vi "T03 - вкл-откл каналов(Base Functions).vi"() -> ()   [LabVIEW 2009]
uses:
  Z210/Z210 CTL Lib.llb/Z210 CTL ADC Inputs Status.ctl
  Z210/Z210 CTL Lib.llb/Z210 CTL ADC Channel Type.ctl
  Z210/Z210 CTL Lib.llb/Z210 CTL DAC Inputs Status.ctl
  Z210/Z210 CTL Lib.llb/Z210 CTL ADC or DAC Function.ctl
  Instance           3 46Saved   T03 - вкл-откл каналов(Base Functions) .vi
  Z210/Z210 Base Functions.llb/Z210 CHANNEL AD Set On/Off.vi
  Z210/Z210 Base Functions.llb/Z210 CHANNEL AD Get On/Off Status.vi
  <vilib>/Utility/error.llb/DialogType.ctl
panel:
  out "Leads Status DAC":T1
  out "Leads Status ADC":T2
  out "leadsAmount DAC":i32
  out "leadsAmount ADC":i32
  out "error out":errorcluster {"code" format="%x"}
  out "workChannel DAC":i32
  out "workChannel ADC":i32
  # "Пример не очень правильной работы с \"канальными\" функциями. Более правильная в T04.\n\na. Выводы АЦП образуют канал работающий в дифференциальном режиме только парами четный-нечетный (нумерацию с 0).\nНапример выводы №0 и №1 могут работать в дифференциальном режиме, а №1 и №2 — нет.\nb. Если опросить состояние выводов АЦП, работающих в дифференциальном режиме, то будет как на Рис 1. Вне зависимости\nбыл ли включен нечетный канал явно, он будет отмечен как выключенный (ср. T03 и T04).\nс. При использовании Base Function легко допустить ошибку (см. п3)."
  # "Рис. 1"
  # "нельзя проверить правильно ли работает этот пример пока нет сбора данных."
  # "Общее число каналов в устройстве"
  # "Количество включенных каналов"
  # "Программа отключает все каналы (подтверждение),\nзатем предлагает включить последовательно несколько\nсначала синфазных, а затем дифференциальных каналов\n\n1. Синфазные каналы включаются корректно в любом количестве\nне превышающем число выводов.\n2. Если количестов синфазных каналов четное — дифф тоже\nвключаются норм.\n3. Внимание! Попытка включить в синфазном режиме 0й и\nв дифференциальном 1й и 2й выводы не приведет к ошибке,\nкак можно было бы ожидать. Вместо этого дифференциальный \nканал образуют 0й и 1й выводы, а состояние 2го зависит\nот того как включать, и что с ним было до того. (ср. T04)"
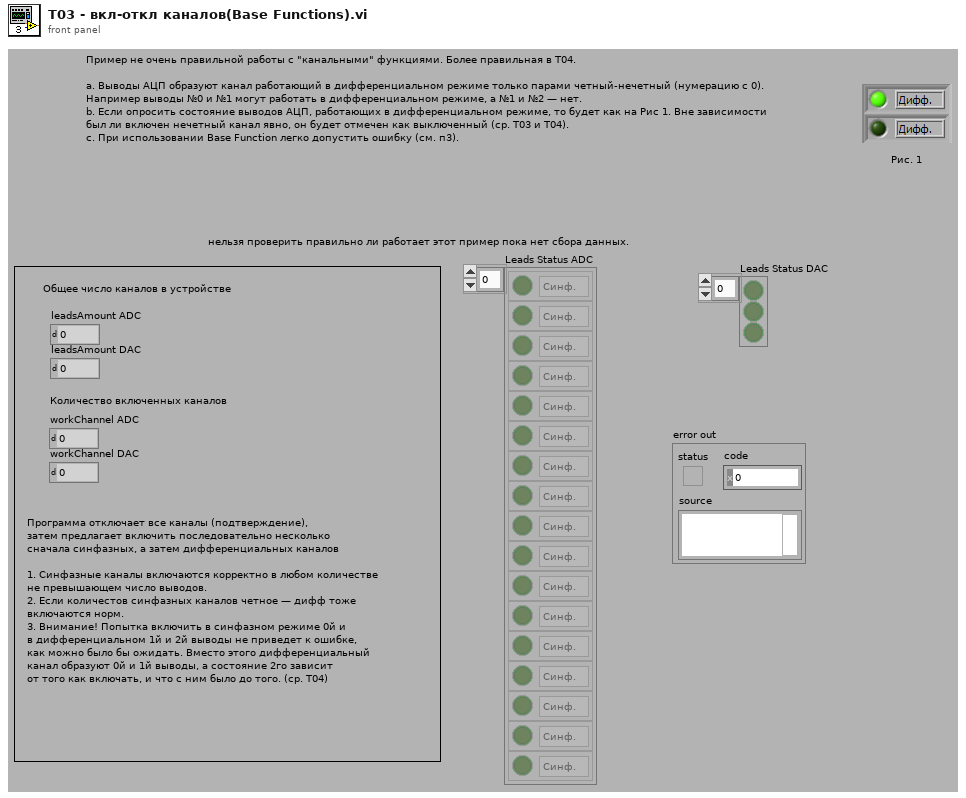
[diagram p1: front panel]
types:
  T1 = typedef "Z210 CTL DAC Inputs Status.ctl" = bool[]
  T2 = typedef "Z210 CTL ADC Inputs Status.ctl" = cluster{"isEnabled?":bool, "ADCchType":T3}[]
  T3 = typedef "Z210 CTL ADC Channel Type.ctl" = enum16{"Синф.", "Дифф."}
  T4 = typedef "Z210 CTL ADC or DAC Function.ctl" = enum16{"АЦП", "ЦАП", "Both"}
  T5 = typedef "Z210 CTL Unit Data .ctl" = cluster{"typeDevice":i32, "numberDSP":i32}
  T6 = typedef "DialogType.ctl" = u16
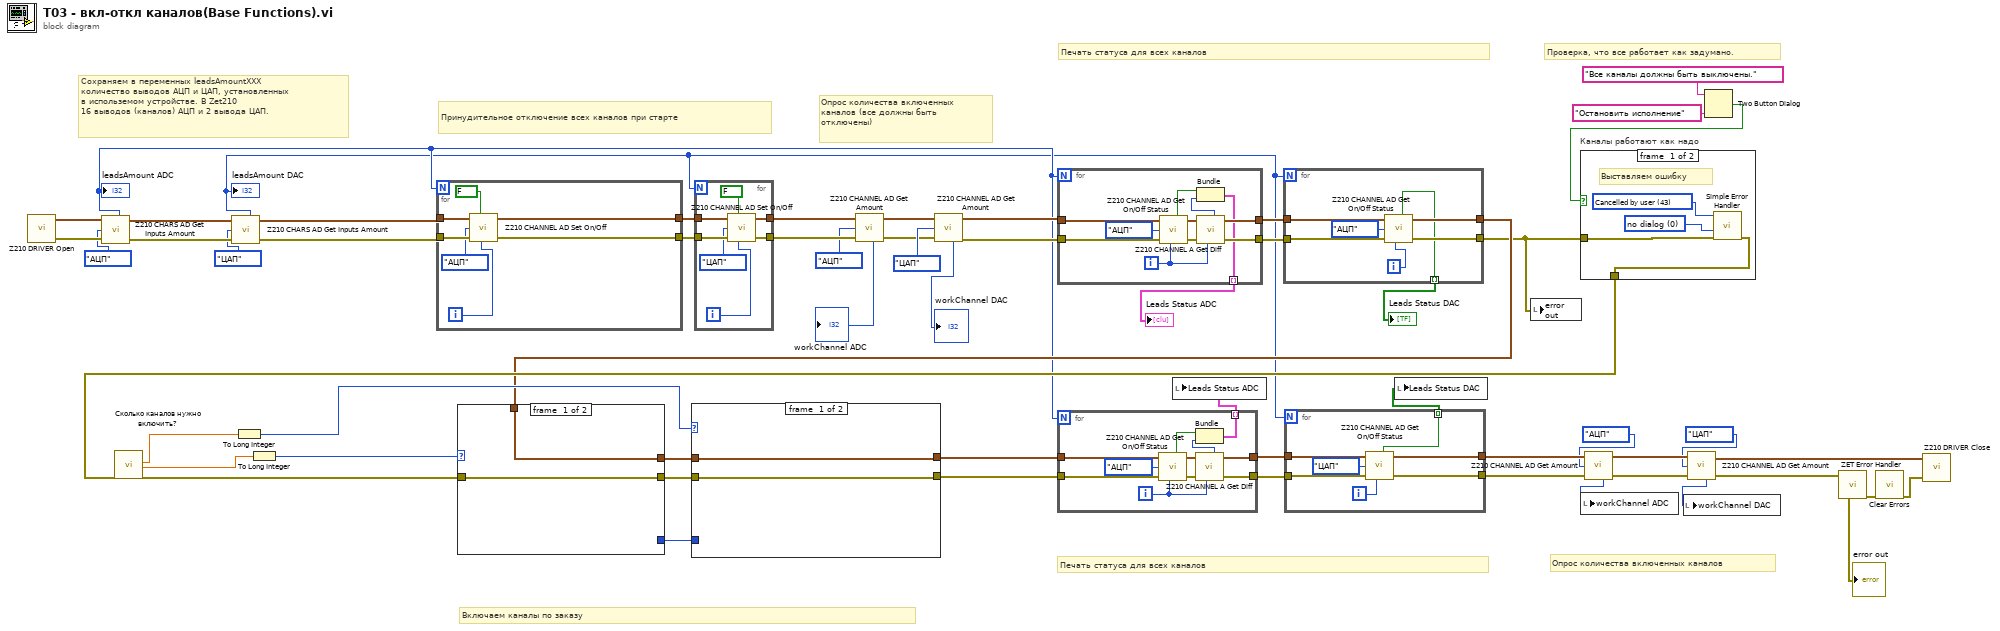
[diagram p0: block diagram]
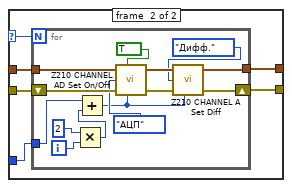
[diagram p2: hidden frame]
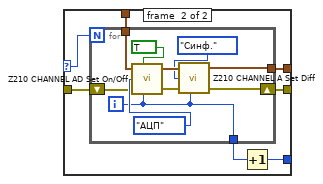
[diagram p3: hidden frame]
diagram:
  # "Сохраняем в переменных leadsAmountXXX\nколичество выводов АЦП и ЦАП, установленных\nв использемом устройстве. В Zet210 \n16 выводов (каналов) АЦП и 2 вывода ЦАП."
  # "Опрос количества включенных каналов"
  # "Печать статуса для всех каналов"
  # "Включаем каналы по заказу"
  # "Проверка, что все работает как задумано."
  # "Печать статуса для всех каналов"
  # "Опрос количества включенных\nканалов (все должны быть\nотключены)"
  # "Принудительное отключение всех каналов при старте"
  n1 = call "Z210 DRIVER Open.vi"() -> ("unitData out"=w32:T5, "error IO"=w33:errorcluster)  [unwired: 8 in]
  n2 = call "Z210 CHARS AD Get Inputs Amount.vi"("unitData in"=w32, "AorD"=Z210_CTL_ADC_or_DAC_Function."АЦП", "error in (no error)"=w33) -> ("inputsAmount"=w2:i32, "unitData out"=w5:T5, "error out"=w4:errorcluster)  [unwired: 4 in]
  "leadsAmount ADC" <- w2
  n3 = call "Z210 CHARS AD Get Inputs Amount.vi"("unitData in"=w5, "AorD"=Z210_CTL_ADC_or_DAC_Function."ЦАП", "error in (no error)"=w4) -> ("inputsAmount"=w1:i32, "unitData out"=w30:T5, "error out"=w31:errorcluster)  [unwired: 4 in]
  "leadsAmount DAC" <- w1
  n4 = for {
    N: w2 -> [_]
    tunnel: w31 -> [w65]
    tunnel: [w60] -> w54
    tunnel: w30 -> [w63]
    tunnel: [w61] -> w55
    i -> [w62]
    n5 = call "Z210 CHANNEL AD Set On/Off.vi"("unitData in"=w63, "enable?"=FALSE, "AorD"=Z210_CTL_ADC_or_DAC_Function."АЦП", "error in (no error)"=w65, "inputNumber"=w62) -> ("unitData out"=w61:T5, "error out"=w60:errorcluster)  [unwired: 3 in]
  }
  n6 = for {
    N: w1 -> [_]
    tunnel: w54 -> [w72]
    tunnel: [w69] -> w39
    tunnel: w55 -> [w68]
    tunnel: [w67] -> w40
    i -> [w70]
    n7 = call "Z210 CHANNEL AD Set On/Off.vi"("unitData in"=w68, "enable?"=FALSE, "AorD"=Z210_CTL_ADC_or_DAC_Function."ЦАП", "error in (no error)"=w72, "inputNumber"=w70) -> ("unitData out"=w67:T5, "error out"=w69:errorcluster)  [unwired: 3 in]
  }
  n8 = call "Z210 CHANNEL AD Get Amount.vi"("unitData in"=w40, "AorD"=Z210_CTL_ADC_or_DAC_Function."АЦП", "error in (no error)"=w39) -> ("unitData out"=w42:T5, "activeChannelsAmount"=→"workChannel ADC":i32, "error out"=w41:errorcluster)  [unwired: 4 in]
  n9 = call "Z210 CHANNEL AD Get Amount.vi"("unitData in"=w42, "AorD"=Z210_CTL_ADC_or_DAC_Function."ЦАП", "error in (no error)"=w41) -> ("unitData out"=w38:T5, "activeChannelsAmount"=→"workChannel DAC":i32, "error out"=w37:errorcluster)  [unwired: 4 in]
  n10 = for {
    N: w2 -> [_]
    tunnel: w38 -> [w83]
    tunnel: w37 -> [w82]
    tunnel: [w77] -> w53
    tunnel: [w78] -> w52
    tunnel: [w74] -> w29 mode=indexing
    i -> [w76]
    n11 = call "Z210 CHANNEL AD Get On/Off Status.vi"("unitData in"=w83, "AorD"=Z210_CTL_ADC_or_DAC_Function."АЦП", "error in (no error)"=w82, "inputNumber"=w76) -> ("isEnabled?"=w75:bool, "unitData out"=w80:T5, "error out"=w79:errorcluster)  [unwired: 3 in]
    n12 = call "Z210 CHANNEL A Get Diff.vi"("unitData in"=w80, "error in (no error)"=w79, "inputNumber"=w76) -> ("ADCchType"=w73:T3, "unitData out"=w77:T5, "error out"=w78:errorcluster)  [unwired: 4 in]
    n13 = Bundle("isEnabled?"=w75, "ADCchType"=w73) -> (w74:cluster{"isEnabled?":bool, "ADCchType":T3})  [unwired: 1 in]
  }
  "Leads Status ADC" <- w29
  n14 = for {
    N: w1 -> [_]
    tunnel: [w88] -> w25
    tunnel: [w87] -> w22
    tunnel: [w86] -> w28 mode=indexing
    tunnel: w53 -> [w85]
    tunnel: w52 -> [w84]
    i -> [w90]
    n15 = call "Z210 CHANNEL AD Get On/Off Status.vi"("unitData in"=w85, "AorD"=Z210_CTL_ADC_or_DAC_Function."АЦП", "error in (no error)"=w84, "inputNumber"=w90) -> ("isEnabled?"=w86:bool, "unitData out"=w88:T5, "error out"=w87:errorcluster)  [unwired: 3 in]
  }
  "Leads Status DAC" <- w28
  n16 = local write "error out"(w22) -> ()
  n17 = Two Button Dialog(message="Все каналы должны быть выключены.", 1:"Остановить исполнение" ("F button name (\"Cancel\")")) -> (T button?=w21:bool)  [unwired: 1 in]
  n18 = case "Каналы работают как надо" shown="False" w21 {
    tunnel: [w93 w95] -> w51
    tunnel: w22 -> [w94 w95]
    frame #0 {
      w92 = T6 0 items=["no dialog", "OK message", "continue or stop message", "OK message + warnings", "continue/stop + warnings"] ("type of dialog (OK msg:1)")
      w91 = 43 items=["No error", "Argument error", "Memory is full", "Out of zone", "End of file", "File already open", "Generic file I/O error", "File not found", "File permission error", "Disk is full", "Duplicate path", "Too many files open", "System feature not enabled", "Resource file not found", "Cannot add resource", "Resource not found", "Image not found", "Image memory error", "Pen does not exist", "Config type invalid", "Config token not found", "Config parse error", "Config memory error", "Bad external code format", "Bad external code offset", "External code not present", "Null window", "Destroy window error", "Null menu", "Print aborted", "Bad print record", "Print driver error", "Windows error during printing", "Memory error during printing", "Print dialog error", "Generic print error", "Invalid device refnum", "Device not found", "Device parameter error", "Device unit error", "Cannot open device", "Device call aborted", "Generic error", "Cancelled by user", "Object ID too low", "Object ID too high", "Object not in heap", "Unknown heap", "Unknown object (invalid DefProc)", "Unknown object (DefProc not in table)", "Message out of range", "Invalid (null) method", "Unknown message", "Manager call not supported", "Bad address", "Network operation in progress", "Network operation timed out", "Connection is busy", "Network attribute not supported", "Network error", "Address in use", "System out of memory", "Connection aborted", "Connection refused", "Not connected", "Already connected", "Connection closed", "Initialization error (interapplication manager)", "Bad occurrence", "Wait on unbound occurrence handler", "Occurrence queue overflow", "Datalog type conflict", "Unused", "Unrecognized type (interapplication manager)", "Memory corrupt", "Failed to make temporary DLL", "Old CIN version", "Drag socket not found", "Failed to load drop-object", "Failed to register OLE object", "Failed to release OLE object", "Format specifier type mismatch", "Unknown format specifier", "Too few format specifiers", "Too many format specifiers", "Scan failed", "Newer CIN version", "Error converting to variant", "Runtime menu error", "Password tampered", "Variant attribute not found", "Incompatible variant data type", "Event data is not available", "Event Store is not present", "Occurrence is not found", "Event Queue is not created", "Event info is not available in the type library", "Refnum passed is NULL", "Error retrieving Class GUID", "Error retrieving CoClass GUID", "Error retrieving TypeLib GUID.", "Bad built application magic bytes.", "Specific driver is different from the specific driver associated with the Logical Name.", "There is no session opened to the class driver.", "Max Error", "MAX - Error with config objects", "MAX - Error loading configuration", "MAX - Group not supported", "Singlecast connections can not send to multicast addresses.", "Multicast connections can not send to singlecast addresses.", "Specified IP address not in multicast address range.", "Attempt to write to read-only multicast connection.", "Attempt to read from write-only multicast connection.", "The buffer used to receive a datagram was smaller than the datagram itself"]
      # "Выставляем ошибку"
      n19 = call <vilib>:"Simple Error Handler.vi"("error code (no error:0)"=w91, "type of dialog (OK msg:1)"=w92, "error in (no error)"=w94) -> ("error out"=w93:errorcluster)  [unwired: 2 in, 4 out]
    }
    frame #1 {
    }
  }
  n20 = call "Сколько каналов нужно включить?"("error in (no error)"=w51) -> ("дифференциальных"=w9:dbl, "синфазных"=w10:dbl, "error out"=w57:errorcluster)  [unwired: 15 in, 1 out]
  n21 = To Long Integer(number=w9) -> (32bit integer=w44:i32)
  n22 = To Long Integer(number=w10) -> (32bit integer=w45:i32)
  n23 = case shown="Default" w45 {
    selector: w45 -> [_ w98]
    tunnel: [w97 w104] -> w58
    tunnel: w57 -> [w96 w103]
    tunnel: [w96 w101] -> w56
    tunnel: [_ w100] -> w46
    tunnel: w25 -> [w97 w99]
    frame #0 {
    }
    frame #1 {
      n24 = for {
        N: w98 -> [_]
        tunnel: [w109] -> w102
        tunnel: [w111] -> w104
        tunnel: w99 -> [w113]
        shift-right: [w105] -> w101
        shift-left: w103 -> [w106]
        i -> [w109]
        n25 = call "Z210 CHANNEL AD Set On/Off.vi"("unitData in"=w113, "enable?"=TRUE, "AorD"=Z210_CTL_ADC_or_DAC_Function."АЦП", "error in (no error)"=w106, "inputNumber"=w109) -> ("unitData out"=w112:T5, "error out"=w107:errorcluster)  [unwired: 3 in]
        n26 = call "Z210 CHANNEL A Set Diff.vi"("unitData in"=w112, "ADCchType"=Z210_CTL_ADC_Channel_Type."Синф.", "error in (no error)"=w107, "inputNumber"=w109) -> ("unitData out"=w111:T5, "error out"=w105:errorcluster)  [unwired: 4 in]
      }
      n27 = Increment(x=w102) -> (x+1=w100:i32)
    }
  }
  n28 = case shown="Default" w44 {
    selector: w44 -> [_ w117]
    tunnel: w58 -> [w116 w122]
    tunnel: w56 -> [w115 w121]
    tunnel: [w116 w120] -> w48
    tunnel: [w115 w119] -> w47
    tunnel: w46 -> [_ w118]
    frame #0 {
    }
    frame #1 {
      n29 = for {
        N: w117 -> [_]
        tunnel: w122 -> [w136]
        tunnel: w118 -> [w124]
        tunnel: [w128] -> w120
        shift-right: [w127] -> w119
        shift-left: w121 -> [w134]
        i -> [w126]
        n30 = Multiply(x=2, y=w126) -> (x*y=w123:i32)
        n31 = Add(x=w124, y=w123) -> (x+y=w129:i32)
        n32 = call "Z210 CHANNEL AD Set On/Off.vi"("unitData in"=w136, "enable?"=TRUE, "AorD"=Z210_CTL_ADC_or_DAC_Function."АЦП", "error in (no error)"=w134, "inputNumber"=w129) -> ("unitData out"=w132:T5, "error out"=w130:errorcluster)  [unwired: 3 in]
        n33 = call "Z210 CHANNEL A Set Diff.vi"("unitData in"=w132, "ADCchType"=Z210_CTL_ADC_Channel_Type."Дифф.", "error in (no error)"=w130, "inputNumber"=w129) -> ("unitData out"=w128:T5, "error out"=w127:errorcluster)  [unwired: 4 in]
      }
    }
  }
  n34 = for {
    N: w2 -> [_]
    tunnel: w48 -> [w147]
    tunnel: w47 -> [w146]
    tunnel: [w141] -> w49
    tunnel: [w142] -> w50
    tunnel: [w137] -> w27 mode=indexing
    i -> [w140]
    n35 = call "Z210 CHANNEL AD Get On/Off Status.vi"("unitData in"=w147, "AorD"=Z210_CTL_ADC_or_DAC_Function."АЦП", "error in (no error)"=w146, "inputNumber"=w140) -> ("isEnabled?"=w139:bool, "unitData out"=w144:T5, "error out"=w143:errorcluster)  [unwired: 3 in]
    n36 = call "Z210 CHANNEL A Get Diff.vi"("unitData in"=w144, "error in (no error)"=w143, "inputNumber"=w140) -> ("ADCchType"=w138:T3, "unitData out"=w141:T5, "error out"=w142:errorcluster)  [unwired: 4 in]
    n37 = Bundle("isEnabled?"=w139, "ADCchType"=w138) -> (w137:cluster{"isEnabled?":bool, "ADCchType":T3})  [unwired: 1 in]
  }
  n38 = local write "Leads Status ADC"(w27) -> ()
  n39 = for {
    N: w1 -> [_]
    tunnel: [w152] -> w20
    tunnel: [w151] -> w19
    tunnel: [w150] -> w26 mode=indexing
    tunnel: w49 -> [w149]
    tunnel: w50 -> [w148]
    i -> [w154]
    n40 = call "Z210 CHANNEL AD Get On/Off Status.vi"("unitData in"=w149, "AorD"=Z210_CTL_ADC_or_DAC_Function."ЦАП", "error in (no error)"=w148, "inputNumber"=w154) -> ("isEnabled?"=w150:bool, "unitData out"=w152:T5, "error out"=w151:errorcluster)  [unwired: 3 in]
  }
  n41 = local write "Leads Status DAC"(w26) -> ()
  n42 = call "Z210 CHANNEL AD Get Amount.vi"("unitData in"=w20, "AorD"=Z210_CTL_ADC_or_DAC_Function."АЦП", "error in (no error)"=w19) -> ("unitData out"=w16:T5, "activeChannelsAmount"=w17:i32, "error out"=w15:errorcluster)  [unwired: 4 in]
  n43 = local write "workChannel ADC"(w17) -> ()
  n44 = call "Z210 CHANNEL AD Get Amount.vi"("unitData in"=w16, "AorD"=Z210_CTL_ADC_or_DAC_Function."ЦАП", "error in (no error)"=w15) -> ("unitData out"=w13:T5, "activeChannelsAmount"=w11:i32, "error out"=w14:errorcluster)  [unwired: 4 in]
  "error out" <- w14
  n45 = local write "workChannel DAC"(w11) -> ()
  n46 = call "ZET Error Handler.vi"("error in (no error)"=w14) -> ("error out"=w8:errorcluster)  [unwired: 9 in, 1 out]
  n47 = call <vilib>:"Clear Errors.vi"("error in (no error)"=w8) -> ("error out"=w7:errorcluster)  [unwired: 6 in]
  n48 = call "Z210 DRIVER Close.vi"("unitData in"=w13, "error in (no error)"=w7) -> ()  [unwired: 6 in, 2 out]
